vi "First Step.vi"(8 "error in (no error)":errorcluster, 11 "SQL Statement in":refnum<class "SQL Statement.lvclass">) -> (0 "error out":errorcluster, 2 "Row returned":bool, 3 "SQL Statement out":refnum<class "SQL Statement.lvclass">)   [LabVIEW 2013, in "SQLiteSupport.lvlib" / "SQL Statement.lvclass"]
doc: "Executes a prepared SQL statement."
uses:
  SQL Statement.lvclass
  SQL Statement.lvclass/SQL Statement.ctl
  Error Message.vi
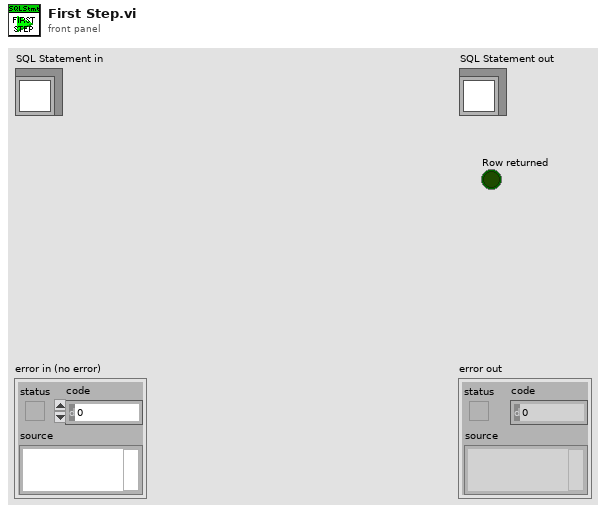
[diagram p1: front panel]
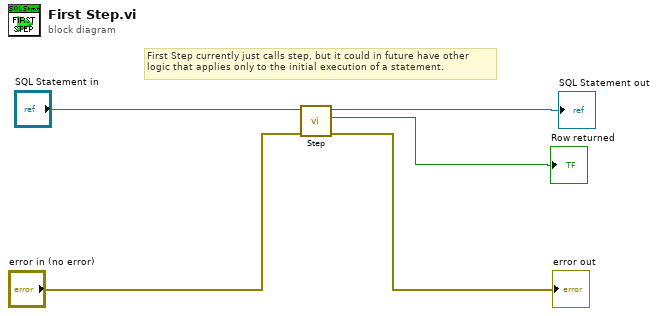
[diagram p0: block diagram]
diagram:
  # "First Step currently just calls step, but it could in future have other \nlogic that applies only to the initial execution of a statement."
  n1 = call "Step.vi"("error in (no error)"="error in (no error)", "SQL Statement in"="SQL Statement in") -> ("error out"=→"error out":errorcluster, "Row returned"=→"Row returned":bool, "SQL Statement out"=→"SQL Statement out":refnum<class "SQL Statement.lvclass">)  [unwired: 7 in]
